vi "lecture1-a.vi"() -> ()   [LabVIEW 2014]
panel:
  out "Area (cm^2)":dbl format="%#_13g"
  in  "Base (cm)":dbl format="%#_13g"
  in  "Height (cm)":dbl format="%#_13g"
  # "Area of a Triangle"
  # "<----------Height----------------->"
  # "<----------Base----------->"
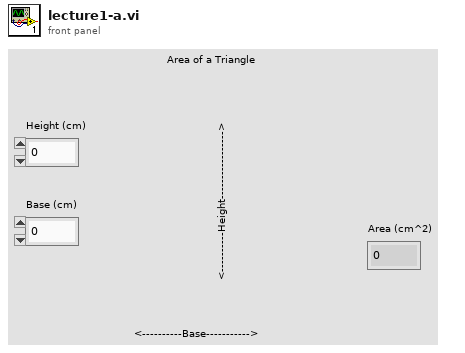
[diagram p1: front panel]
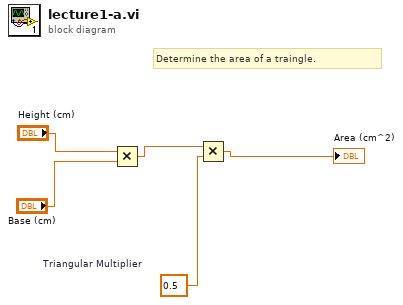
[diagram p0: block diagram]
diagram:
  w2 = 0.5  # Triangular Multiplier
  # "Determine the area of a traingle."
  n1 = Multiply(x="Height (cm)", y="Base (cm)") -> (x*y=w3:dbl)
  n2 = Multiply(x=w3, y=w2) -> (x*y=→"Area (cm^2)":dbl)
